vi "Read Power On Time.vi"(8 "error in (no error)":errorcluster, 11 "MKS MW in":refnum<class "PL MKS MW.lvclass">) -> (0 "error out":errorcluster, 2 "power on time, s":u32 format="%<%H:%M:%S>t", 3 "MKS MW out":refnum<class "PL MKS MW.lvclass">)   [LabVIEW 2015, in "PL MKS MW.lvclass"]
doc: "Reads device power on time."
uses:
  PL MKS MW.lvclass
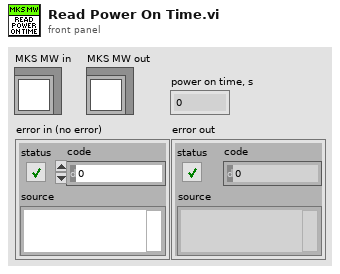
[diagram p1: front panel]
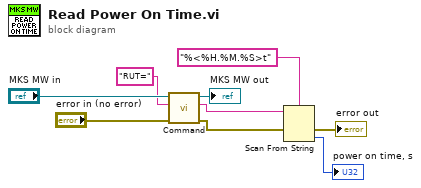
[diagram p0: block diagram]
diagram:
  n1 = call "Command.vi"("error in (no error)"="error in (no error)", "command"="RUT=", "MKS MW in"="MKS MW in") -> ("error out"=w5:errorcluster, "response data"=w3:string, "MKS MW out"=→"MKS MW out":refnum<class "PL MKS MW.lvclass">)  [unwired: 6 in]
  n2 = Scan From String(format string="%<%H.%M.%S>t", input string=w3, error in=w5) -> (error out=→"error out":errorcluster, output 1=→"power on time, s":u32)  [unwired: 2 in, 2 out]
